vi "Set PID.vi"(5 "Output #":i32=1, 6 "D":dbl, 7 "P manual":dbl, 8 "error in (no error)":errorcluster, 9 "I":dbl, 10 "P":dbl, 11 "Temperature Controller Driver in":refnum<class "Temperature Controller Driver.lvclass">) -> (0 "error out":errorcluster, 3 "Temperature Controller Driver out":refnum<class "Temperature Controller Driver.lvclass">)   [LabVIEW 2021, in "Temperature Controller Driver.lvclass"]
uses:
  Temperature Controller Driver.lvclass
  Temperature Controller Driver.lvclass/Temperature Controller Driver.ctl
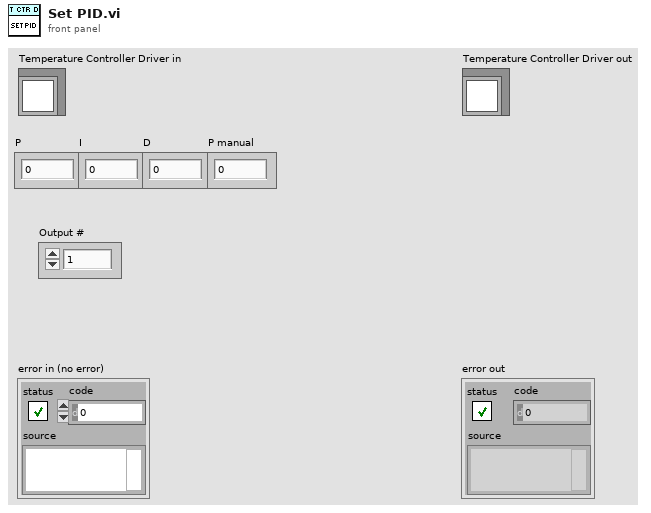
[diagram p1: front panel]
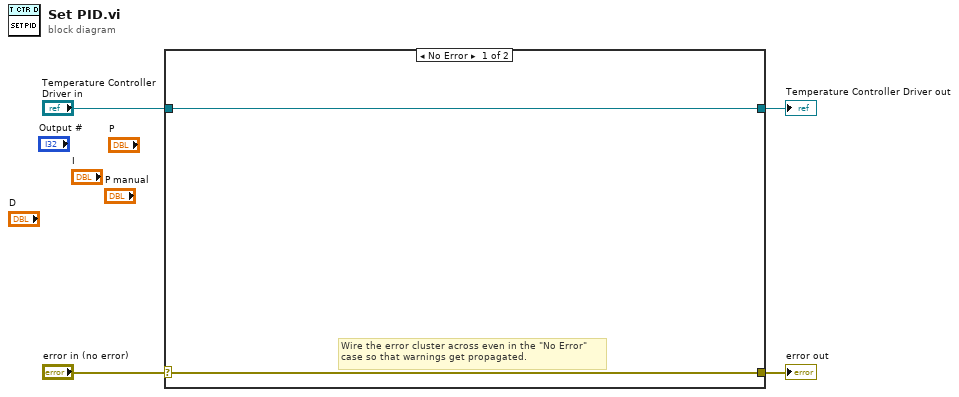
[diagram p0: block diagram]
diagram:
  n1 = case shown="No Error" "error in (no error)" {
    selector: "error in (no error)" -> [w5 w8]
    tunnel: [w5 w8] -> w3
    tunnel: [w6 w7] -> w1
    tunnel: "Temperature Controller Driver in" -> [w6 w7]
    frame No Error {
      # "Wire the error cluster across even in the \"No Error\"\ncase so that warnings get propagated."
    }
    frame Error {
    }
  }
  "error out" <- w3
  "Temperature Controller Driver out" <- w1
